vi "db_test.vi"   [LabVIEW 2015]
uses:
  C:/Users/Arkadiusz/SkyDrive/Dokumenty/Visual Studio 2015/Projects/NordicDatabaseDLL/NordicDatabaseDLL/bin/Debug/NordicDatabaseDLL.dll
  SkyDrive/Dokumenty/Visual Studio 2015/Projects/NordicDatabaseDLL/NordicDatabaseDLL/bin/Debug/NordicDatabaseDLL.dll
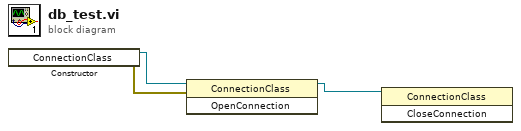
[diagram p0: block diagram]
diagram:
  n1 = constructor class="ConnectionClass"() -> (reference out=w3:refnum<k24>, error out=w2:errorcluster)  [unwired: 3 in, 1 out]
  n2 = invoke class="ConnectionClass" method="OpenConnection"(reference=w3, error in=w2) -> (reference out=w1:refnum<k24>)  [unwired: 1 in, 2 out]
  n3 = invoke class="ConnectionClass" method="CloseConnection"(reference=w1) -> ()  [unwired: 2 in, 3 out]
